vi "Insertion Jig Pick Point.vi"(11 "error in":errorcluster) -> (3 "error out":errorcluster)   [LabVIEW 2013]
uses:
  ROS/Code/SubVIs/BaxterCamera.ctl
  <vilib>/Analysis/baseanly.llb/Mean (DBL).vi
  <vilib>/Analysis/NI_AALBase.lvlib
panel:
  out "Y shift":dbl format="%0.2f"
  out "X shift":dbl
  in  "Camera":T1=enum."right_hand_camera"
  in  "Jig Pick Image":picture
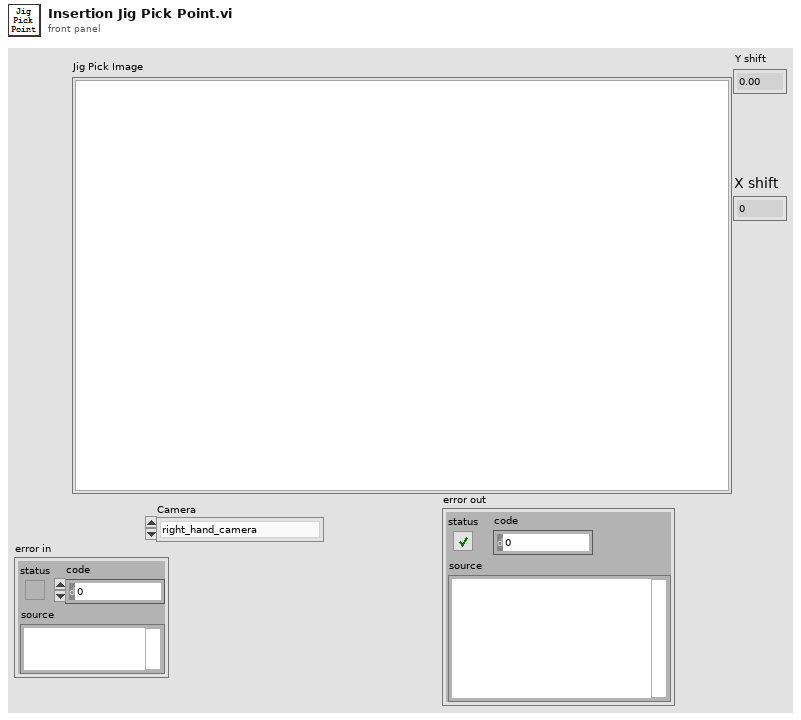
[diagram p1: front panel]
types:
  T1 = typedef "BaxterCamera.ctl" = enum16{"left_hand_camera", "right_hand_camera", "head_camera"}
  T2 = cluster{"X":dbl, "Y":dbl, "Z":dbl, "O":dbl, "A":dbl, "T":dbl}
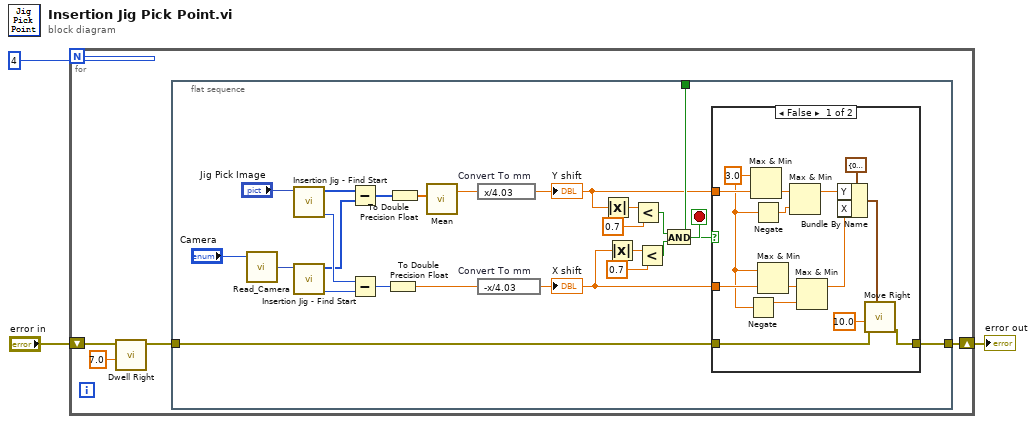
[diagram p0: block diagram]
diagram:
  n1 = for {
    N: 4 -> [_]
    shift-right: [w7] -> w1
    shift-left: "error in" -> [w5]
    stop <- w8 stop-if-true
    n2 = call "Dwell Right.vi"("Wait Time"=7.0, "error in"=w5) -> ("error out"=w4:errorcluster)  [unwired: 9 in]
    n3 = flat-sequence {
      tunnel: [w12] -> w8
      tunnel: w4 -> [w10]
      tunnel: [w9] -> w7
      frame #0 {
        n4 = call "Read_Camera.vi"("Camera"="Camera") -> ("picture"=w29:picture)  [unwired: 4 in, 2 out]
        n5 = call "Insertion Jig - Find Start.vi"("picture"="Jig Pick Image") -> ("First Column"=w26:i32, "Edge Set"=w24:i32[])  [unwired: 9 in]
        n6 = call "Insertion Jig - Find Start.vi"("picture"=w29) -> ("First Column"=w28:i32, "Edge Set"=w25:i32[])  [unwired: 9 in]
        n7 = Subtract(x=w24, y=w25) -> (x-y=w23:i32[])
        n8 = Subtract(x=w26, y=w28) -> (x-y=w27:i32)
        n9 = To Double Precision Float(number=w27) -> (double precision float=w11:dbl)
        n10 = To Double Precision Float(number=w23) -> (double precision float=w22:dbl[])
        n11 = call-poly <vilib>:"Mean.vi"("X"=w22) -> ("mean"=w21:dbl)  [unwired: 1 out]
        n12 = expression code="x/4.03" "Convert To mm"(w21) -> (w15:dbl)
        "Y shift" <- w15
        n13 = expression code="-x/4.03" "Convert To mm"(w11) -> (w20:dbl)
        "X shift" <- w20
        n14 = Absolute Value(x=w15) -> (abs(x)=w17:dbl)
        n15 = Absolute Value(x=w20) -> (abs(x)=w19:dbl)
        n16 = Less?(x=w17, y=0.7) -> (x < y?=w14:bool)
        n17 = Less?(x=w19, y=0.7) -> (x < y?=w13:bool)
        n18 = And(x=w14, y=w13) -> (x .and. y?=w12:bool)
        n19 = case shown="False" w12 {
          tunnel: w20 -> [w38 _]
          tunnel: w15 -> [w41 _]
          tunnel: w10 -> [w36 w46]
          tunnel: [w32 w46] -> w9
          frame False {
            w33 = 3.0 ("x")
            n20 = Negate(x=w33) -> (-x=w34:dbl)
            n21 = Max & Min(x=w33, y=w41) -> (min(x,y)=w42:dbl)  [unwired: 1 out]
            n22 = Negate(x=w33) -> (-x=w35:dbl)
            n23 = Max & Min(x=w33, y=w38) -> (min(x,y)=w39:dbl)  [unwired: 1 out]
            n24 = Max & Min(x=w42, y=w35) -> (max(x,y)=w40:dbl)  [unwired: 1 out]
            n25 = Max & Min(x=w39, y=w34) -> (max(x,y)=w37:dbl)  [unwired: 1 out]
            n26 = Bundle By Name(cluster=T2 {"X"=0.0, "Y"=0.0, "Z"=0.0, "O"=0.0, "A"=0.0, "T"=0.0} ("Goal Axes"), "Y"=w40, "X"=w37) -> (w44:T2)
            n27 = call "Move Right.vi"("Goal Axes"=w44, "error in"=w36, "Speed"=10.0) -> ("error out"=w32:errorcluster)  [unwired: 4 in, 4 out]
          }
          frame True {
          }
        }
      }
    }
  }
  "error out" <- w1
